vi "test_libssh2_channel_request_pty_size_ex.vi"() -> ()   [LabVIEW 2013, in "libssh2_integration_tests.lvlib"]
uses:
  libssh2_integration_tests.lvlib
  <vilib>/addons/_JKI Toolkits/Caraya/classes/Test/Test.lvclass
  libssh2/libssh2.lvlib
  <vilib>/addons/_JKI Toolkits/Caraya/classes/Assert/Assert.lvclass
panel:
  out "error out":errorcluster
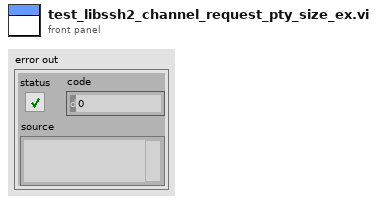
[diagram p1: front panel]
types:
  T1 = typedef "libssh2.lvlib/Session Refnum.ctl" = refnum<k1>
  T2 = typedef "libssh2.lvlib/Channel Refnum.ctl" = refnum<k1>
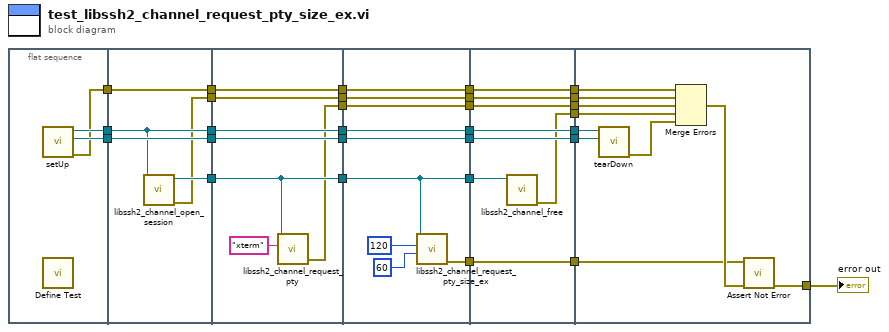
[diagram p0: block diagram]
diagram:
  n1 = flat-sequence {
    tunnel: [w32] -> w29
    tunnel: [w31] -> w28
    tunnel: [w30] -> w20
    tunnel: w29 -> [w36]
    tunnel: w28 -> [w37]
    tunnel: [w36] -> w27
    tunnel: [w37] -> w26
    tunnel: [w35] -> w25
    tunnel: w20 -> [w34]
    tunnel: [w34] -> w19
    tunnel: [w33] -> w17
    tunnel: w27 -> [w44]
    tunnel: w26 -> [w43]
    tunnel: w25 -> [w40]
    tunnel: [w44] -> w14
    tunnel: [w43] -> w12
    tunnel: [w40] -> w10
    tunnel: w19 -> [w42]
    tunnel: [w42] -> w8
    tunnel: w17 -> [w41]
    tunnel: [w41] -> w6
    tunnel: [w38] -> w3
    tunnel: w14 -> [w53]
    tunnel: [w53] -> w13
    tunnel: w12 -> [w52]
    tunnel: [w52] -> w11
    tunnel: w10 -> [w47]
    tunnel: [w47] -> w9
    tunnel: w8 -> [w51]
    tunnel: [w51] -> w7
    tunnel: w6 -> [w50]
    tunnel: [w50] -> w5
    tunnel: [w49] -> w4
    tunnel: w3 -> [w48]
    tunnel: [w48] -> w2
    tunnel: w13 -> [w61]
    tunnel: w11 -> [w60]
    tunnel: w9 -> [w59]
    tunnel: [w61] -> w24
    tunnel: [w60] -> w23
    tunnel: [w58] -> w21
    tunnel: w7 -> [w57]
    tunnel: [w57] -> w18
    tunnel: w5 -> [w56]
    tunnel: [w56] -> w16
    tunnel: w4 -> [w55]
    tunnel: [w55] -> w15
    tunnel: w2 -> [w54]
    tunnel: [w54] -> w1
    tunnel: w24 -> [w71]
    tunnel: w23 -> [w70]
    tunnel: [w69] -> w22
    tunnel: w21 -> [w67]
    tunnel: w18 -> [w66]
    tunnel: w16 -> [w64]
    tunnel: w15 -> [w63]
    tunnel: w1 -> [w62]
    frame #0 {
      n2 = call "setUp.vi"() -> ("error out"=w30:errorcluster, "connection ID"=w31:refnum<k5>, "session"=w32:T1)  [unwired: 9 in]
      n3 = call <vilib>:"Define Test.vi"() -> ()  [unwired: 10 in, 2 out]
    }
    frame #1 {
      n4 = call "libssh2_channel_open_session.vi"("session"=w36) -> ("error out"=w33:errorcluster, "channel"=w35:T2)  [unwired: 9 in]
    }
    frame #2 {
      n5 = call "libssh2_channel_request_pty.vi"("term"="xterm", "channel"=w40) -> ("error out"=w38:errorcluster)  [unwired: 9 in]
    }
    frame #3 {
      n6 = call "libssh2_channel_request_pty_size_ex.vi"("height"=60, "width"=120, "channel"=w47) -> ("error out"=w49:errorcluster)  [unwired: 8 in]
    }
    frame #4 {
      n7 = call "libssh2_channel_free.vi"("channel"=w59) -> ("error out"=w58:errorcluster)  [unwired: 10 in]
    }
    frame #5 {
      n8 = call "tearDown.vi"("connection ID"=w70, "session"=w71) -> ("error out"=w68:errorcluster)  [unwired: 9 in]
      n9 = Merge Errors(w66, w64, w62, w67, w68) -> (w65:errorcluster)
      n10 = call <vilib>:"Assert Not Error.vi"("error in (no error)"=w65, "Not Error?"=w63) -> ("error out"=w69:errorcluster)  [unwired: 8 in, 1 out]
    }
  }
  "error out" <- w22
